vi "GetSampleData.vi"(0 "TCP网络连接输入":refnum<k5>, 5 "Row":dbl, 7 "id":string, 9 "SampleTime":string, 11 "错误输入（无错误）":errorcluster) -> (4 "采样数据":string[][](array[string]), 6 "存在记录？":bool, 15 "错误输出":errorcluster)   [LabVIEW 2014]
uses:
  Global/ClientGlobalCY.vi
panel:
  out "连接的字符串":string
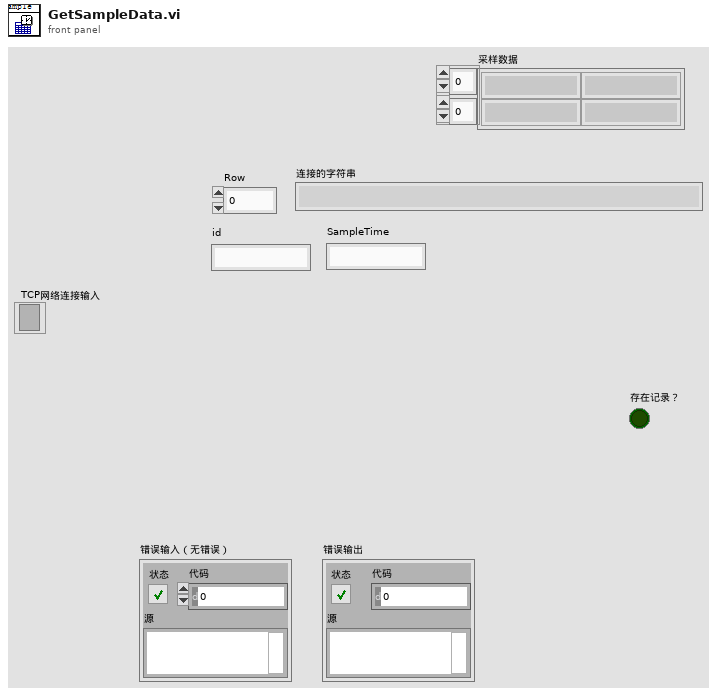
[diagram p1: front panel]
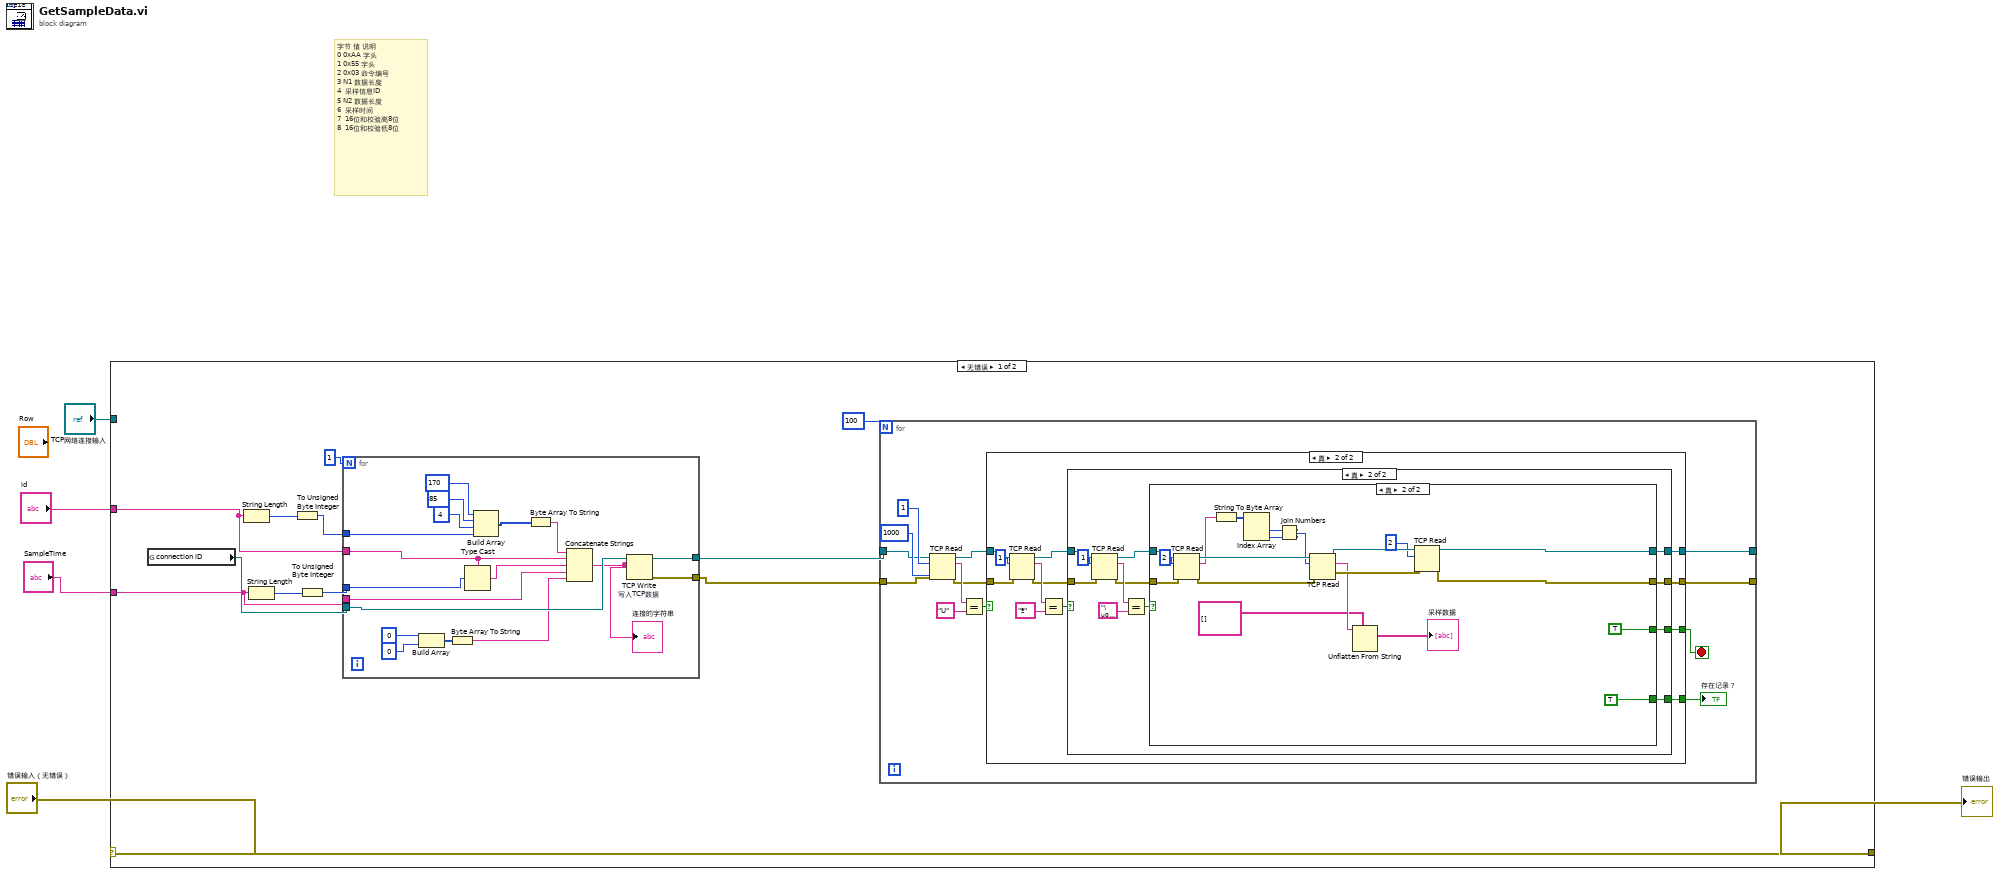
[diagram p0: block diagram]
diagram:
  # "字节\t值\t说明\n0\t0xAA\t字头\n1\t0x55\t字头\n2\t0x03\t命令编号\n3\tN1\t数据长度\n4\t\t采样信息ID\n5\tN2\t数据长度\n6\t\t采样时间\n7\t\t16位和校验高8位\n8\t\t16位和校验低8位"
  n1 = case shown="无错误" "错误输入（无错误）" {
    selector: "错误输入（无错误）" -> [w6 w99]
    tunnel: [w6 w99] -> w5
    tunnel: "TCP网络连接输入" -> [_ _]
    tunnel: "id" -> [w12 _]
    tunnel: "SampleTime" -> [w9 _]
    frame No Error {
      n2 = global read "ClientGlobalCY.vi" "connection ID"() -> (w15:refnum<k5>)
      n3 = String Length(string=w12) -> (length=w14:i32)
      n4 = String Length(string=w9) -> (length=w11:i32)
      n5 = To Unsigned Byte Integer(number=w14) -> (unsigned 8bit integer=w13:u8)
      n6 = To Unsigned Byte Integer(number=w11) -> (unsigned 8bit integer=w10:u8)
      n7 = for {
        N: 1 -> [_]
        tunnel: w15 -> [w96]
        tunnel: [w98] -> w17
        tunnel: w13 -> [w86]
        tunnel: w12 -> [w84]
        tunnel: w10 -> [w85]
        tunnel: w9 -> [w82]
        tunnel: [w97] -> w8
        n8 = Build Array(u8 0, u8 0) -> (w89:u8[])
        n9 = Byte Array To String(unsigned byte array=w89) -> (string=w81:string)
        n10 = Type Cast(type=w84, x=w85) -> (*(type *) &x=w83:string)
        n11 = Build Array(u8 170, u8 85, u8 4, w86) -> (w92:u8[])
        n12 = Byte Array To String(unsigned byte array=w92) -> (string=w88:string)
        n13 = Concatenate Strings(w88, w84, w83, w82, w81) -> (w87:string)
        "连接的字符串" <- w87
        n14 = TCP Write "写入TCP数据"(connection ID=w96, data in=w87) -> (connection ID out=w98:refnum<k5>, error out=w97:errorcluster)  [unwired: 2 in, 1 out]
      }
      n15 = for "For循环" {
        N: 100 -> [_]
        tunnel: w17 -> [w23]
        tunnel: [w20] -> _
        tunnel: w8 -> [w22]
        tunnel: [w18] -> _
        stop <- w21 stop-if-true
        n16 = TCP Read(connection ID=w23, bytes to read=1 ("读取的字节"), error in (no error)=w22, 9:1000 ("超时毫秒(25000)")) -> (connection ID out=w26:refnum<k5>, data out=w28:string, error out=w25:errorcluster)  [unwired: 1 in]
        n17 = Equal?(x=w28, y="U") -> (x = y?=w27:bool)
        n18 = case shown="真" w27 {
          tunnel: w26 -> [w32 w41]
          tunnel: w25 -> [w31 w40]
          tunnel: [w32 w36] -> w20
          tunnel: [w31 w35] -> w18
          tunnel: [_ w34] -> w21
          tunnel: [_ w33] -> w19
          frame False {
          }
          frame True {
            n19 = TCP Read(connection ID=w41, bytes to read=1 ("读取的字节"), error in (no error)=w40) -> (connection ID out=w38:refnum<k5>, data out=w42:string, error out=w37:errorcluster)  [unwired: 2 in]
            n20 = Equal?(x=w42, y="ª") -> (x = y?=w39:bool)
            n21 = case shown="真" w39 {
              tunnel: w38 -> [w46 w55]
              tunnel: w37 -> [w45 w54]
              tunnel: [w46 w50] -> w36
              tunnel: [w45 w49] -> w35
              tunnel: [_ w48] -> w34
              tunnel: [_ w47] -> w33
              frame False {
              }
              frame True {
                n22 = TCP Read(connection ID=w55, bytes to read=1 ("读取的字节"), error in (no error)=w54) -> (connection ID out=w53:refnum<k5>, data out=w56:string, error out=w52:errorcluster)  [unwired: 2 in]
                n23 = Equal?(x=w56, y="\u0004") -> (x = y?=w51:bool)
                n24 = case shown="真" w51 {
                  tunnel: w53 -> [w60 w79]
                  tunnel: w52 -> [w59 w78]
                  tunnel: [w60 w71] -> w50
                  tunnel: [w59 w72] -> w49
                  tunnel: [_ TRUE] -> w48
                  tunnel: [_ TRUE] -> w47
                  frame False {
                  }
                  frame True {
                    n25 = TCP Read(connection ID=w79, bytes to read=2 ("读取的字节"), error in (no error)=w78) -> (connection ID out=w77:refnum<k5>, data out=w62:string, error out=w76:errorcluster)  [unwired: 2 in]
                    n26 = String To Byte Array(string=w62) -> (unsigned byte array=w65:u8[])
                    n27 = Index Array(array=w65) -> (element #1=w64:u8, element #2=w63:u8)  [unwired: 2 in]
                    n28 = Join Numbers(hi=w64, lo=w63) -> ((hi.lo)=w61:u16)
                    n29 = TCP Read(connection ID=w77, bytes to read=w61, error in (no error)=w76) -> (connection ID out=w74:refnum<k5>, data out=w68:string, error out=w73:errorcluster)  [unwired: 2 in]
                    n30 = Unflatten From String(type=string[][] [], binary string=w68) -> (value=→"采样数据":string[][])  [unwired: 3 in, 2 out]
                    n31 = TCP Read(connection ID=w74, bytes to read=2 ("读取的字节"), error in (no error)=w73) -> (connection ID out=w71:refnum<k5>, error out=w72:errorcluster)  [unwired: 2 in, 1 out]
                  }
                }
              }
            }
          }
        }
        "存在记录？" <- w19
      }
    }
    frame Error {
    }
  }
  "错误输出" <- w5
